vi "ConvertSystemDefinitionPropertyTypeToEnum.vi"(8 "error in (no error)":errorcluster, 11 "type":i32) -> (0 "error out":errorcluster, 3 "type":T1)   [LabVIEW 2016, in "VeriStandTestUtilities.lvlib"]
uses:
  VeriStandTestUtilities.lvlib
  SystemDefinitionPropertyType.ctl
panel:
  in  "type enum":T1
  in  "type ring":i32(ring) items=["K_STRING", "K_BOOL", "K_I32", "K_U32", "K_DOUBLE", "K_U64", "K_VARIANT", "K_DEPENDENTFILE", "K_DEPENDENTNODE", "K_DATASOURCENODE", "K_U16", "K_DBLARR", "K_U32ARR", "K_I32ARR", "K_STRINGARR", "K_DICTIONARY", "K_DICTIONARYARR", "K_BINARYSTRING", "K_I16", "K_I64", "K_BOOLARR", "K_U64ARR", "K_U16ARR", "K_I64ARR", "K_I16ARR"]
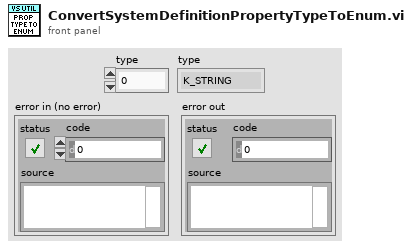
[diagram p1: front panel]
types:
  T1 = typedef "VeriStandTestUtilities.lvlib/SystemDefinitionPropertyType.ctl" = enum16{"K_STRING", "K_BOOL", "K_I32", "K_U32", "K_DOUBLE", "K_U64", "K_VARIANT", "K_DEPENDENTFILE", "K_DEPENDENTNODE", "K_DATASOURCENODE", "K_U16", "K_DBLARR", "K_U32ARR", "K_I32ARR", "K_STRINGARR", "K_DICTIONARY", "K_DICTIONARYARR", "K_BINARYSTRING", "K_I16", "K_I64", "K_BOOLARR", "K_U64ARR", "K_U16ARR", "K_I64ARR", "K_I16ARR"}
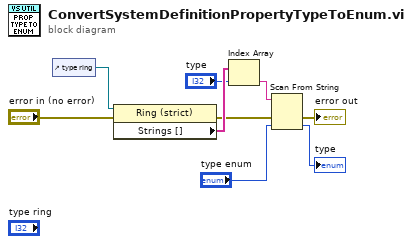
[diagram p0: block diagram]
diagram:
  n1 = control-ref of="type ring"() -> (w9:refnum<vi>)
  n2 = property class="Ring (strict)"(reference=w9, error in="error in (no error)") -> (error out=w3:errorcluster, "Strings []"=w8:string[])  [unwired: 1 out]
  n3 = Index Array(array=w8, index="type") -> (element=w7:string)
  n4 = Scan From String(input string=w7, error in=w3, default 1="type enum") -> (error out=→"error out":errorcluster, output 1=→"type":T1)  [unwired: 2 in, 2 out]
